vi "StressDist_equivalent.vi"(7 "Corrigido":bool, 8 "Error In":errorcluster, 11 "main_FGV_data":T1={"pipe_properties"={"out_radius"=0.0, "in_radius"=0.0, "out_diameter"=0.0, "in_diameter"=0.0, "thickness"=0.0, "inertia"=0.0, "area"=0.0}, "DirPath"=path "L:/Documentos/00 SERVIÇOS/Tensão residual/Olapa 10-2017/Dados/Primeira Seção/Furos", "DirReport"=path "L:/Documentos/00 SERVIÇOS/Tensão residual/Olapa 10-2017/RelatóriosOlapa/Teste", "Points"=[], "ovalization_data"={"AngOval"=[0.0, 60.0, 120.0, 22.5, 45.0, 67.5, 90.0, 112.5, 135.0, 157.5, 180.0], "OvalDiam"=[324.25, 324.6, 324.55, 324.25, 324.55, 324.65, 324.6, 324.65, 324.55, 324.5, 324.4], "Plots"={"Ref"={"X"=[], "Y"=[]}, "Elipse"={"X"=[], "Y"=[]}, "Points"={"X"=[], "Y"=[]}}, "Ampliation"=100.0, "Results"={"MD"=0.0, "mD"=0.0, "Dmed"=0.0, "Oval"=0.0, "ang"=0.0, "X0"=0.0, "Y0"=0.0}}, "StressDist_data"={"Long"={"Plot"=[], "Fit"=[], "ColorMap"=[], "Data"=[], "peirce_data"={"Plot"=[], "Index removidos"=[]}}, "Circ"={"Plot"=[], "Fit"=[], "ColorMap"=[], "Data"=[], "peirce_data"={"Plot"=[], "Index removidos"=[]}}, "Shear"={"Plot"=[], "Fit"=[], "ColorMap"=[], "Data"=[], "peirce_data"={"Plot"=[], "Index removidos"=[]}}, "Equivalent"={"Plot"=[], "Fit"=[], "ColorMap"=[], "Data"=[], "peirce_data"={"Plot"=[], "Index removidos"=[]}}}, "pressure_data"={"Pressure"=[], "StressCircOval"=[], "StressCirc"=[], "StressLong"=[], "Plot"=[], "Angle"=[]}}) -> (0 "Error Out":errorcluster, 3 "main_FGV_data-out":T1={"pipe_properties"={"out_radius"=0.0, "in_radius"=0.0, "out_diameter"=0.0, "in_diameter"=0.0, "thickness"=0.0, "inertia"=0.0, "area"=0.0}, "DirPath"=path "L:/Documentos/00 SERVIÇOS/Tensão residual/Olapa 10-2017/Dados/Primeira Seção/Furos", "DirReport"=path "L:/Documentos/00 SERVIÇOS/Tensão residual/Olapa 10-2017/RelatóriosOlapa/Teste", "Points"=[], "ovalization_data"={"AngOval"=[0.0, 60.0, 120.0, 22.5, 45.0, 67.5, 90.0, 112.5, 135.0, 157.5, 180.0], "OvalDiam"=[324.25, 324.6, 324.55, 324.25, 324.55, 324.65, 324.6, 324.65, 324.55, 324.5, 324.4], "Plots"={"Ref"={"X"=[], "Y"=[]}, "Elipse"={"X"=[], "Y"=[]}, "Points"={"X"=[], "Y"=[]}}, "Ampliation"=100.0, "Results"={"MD"=0.0, "mD"=0.0, "Dmed"=0.0, "Oval"=0.0, "ang"=0.0, "X0"=0.0, "Y0"=0.0}}, "StressDist_data"={"Long"={"Plot"=[], "Fit"=[], "ColorMap"=[], "Data"=[], "peirce_data"={"Plot"=[], "Index removidos"=[]}}, "Circ"={"Plot"=[], "Fit"=[], "ColorMap"=[], "Data"=[], "peirce_data"={"Plot"=[], "Index removidos"=[]}}, "Shear"={"Plot"=[], "Fit"=[], "ColorMap"=[], "Data"=[], "peirce_data"={"Plot"=[], "Index removidos"=[]}}, "Equivalent"={"Plot"=[], "Fit"=[], "ColorMap"=[], "Data"=[], "peirce_data"={"Plot"=[], "Index removidos"=[]}}}, "pressure_data"={"Pressure"=[], "StressCircOval"=[], "StressCirc"=[], "StressLong"=[], "Plot"=[], "Angle"=[]}})   [LabVIEW 2016]
uses:
  MainFGV/main_FGV_data.ctl
  MainFGV/pipe_properties.ctl
  StressCalculations/point_data.ctl
  Ovalization/ovalization_data.ctl
  StressDist_data.ctl
  StressDist_single_data.ctl
  Peirce/peirce_data.ctl
  Pressure/pressure_data.ctl
  StressDist_types.ctl
  Report/report_mods.ctl
panel:
  out "EquiStressCM":dbl[][](graph)
  out "EquiStress":cluster{"X":dbl[], "Y":dbl[]}[](graph) caption="Ovalização"
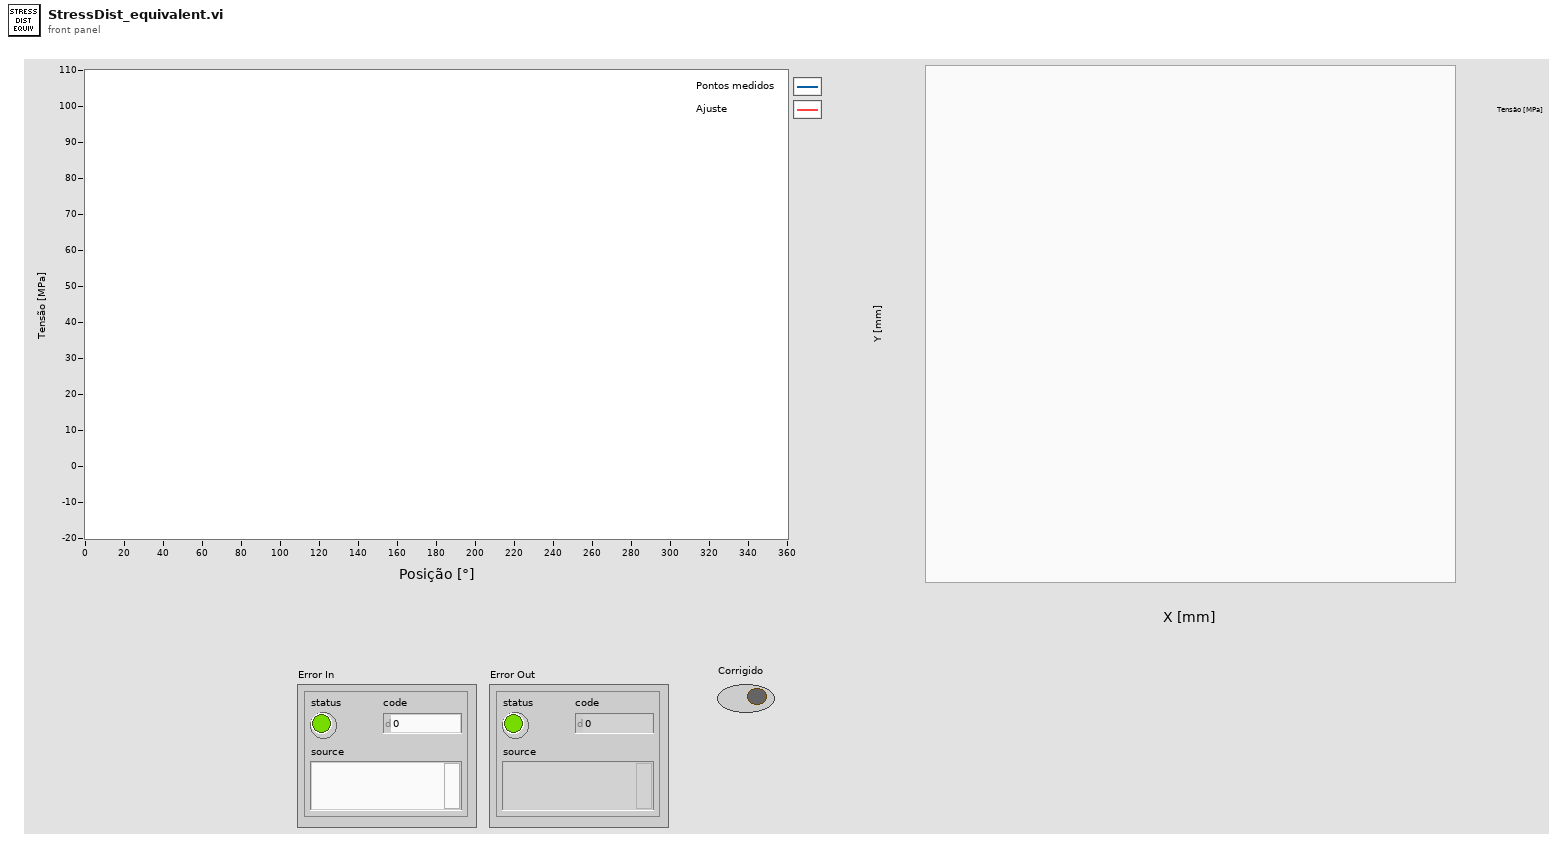
[diagram p1: front panel]
types:
  T1 = typedef "main_FGV_data.ctl" = cluster{"pipe_properties":T2, "DirPath":path, "DirReport":path, "Points":T3[], "ovalization_data":T4, "StressDist_data":T5, "pressure_data":T8}
  T2 = typedef "pipe_properties.ctl" = cluster{"out_radius":dbl, "in_radius":dbl, "out_diameter":dbl, "in_diameter":dbl, "thickness":dbl, "inertia":dbl, "area":dbl}
  T3 = typedef "point_data.ctl" = cluster{"LongStress":dbl, "CircStress":dbl, "ShearStress":dbl, "Pressure":dbl, "Angle":dbl, "Thickness":dbl, "HoleDiam":dbl, "EquiStress":dbl, "S1":dbl, "S2":dbl, "Beta":dbl}
  T4 = typedef "ovalization_data.ctl" = cluster{"AngOval":dbl[], "OvalDiam":dbl[], "Plots":cluster{"Ref":cluster{"X":dbl[], "Y":dbl[]}, "Elipse":cluster{"X":dbl[], "Y":dbl[]}, "Points":cluster{"X":dbl[], "Y":dbl[]}}, "Ampliation":dbl, "Results":cluster{"MD":dbl, "mD":dbl, "Dmed":dbl, "Oval":dbl, "ang":dbl, "X0":dbl, "Y0":dbl}}
  T5 = typedef "StressDist_data.ctl" = cluster{"Long":T6, "Circ":T6, "Shear":T6, "Equivalent":T6}
  T6 = typedef "StressDist_single_data.ctl" = cluster{"Plot":cluster{"Angle":dbl[], "Stress":dbl[]}[], "Fit":dbl[], "ColorMap":dbl[][], "Data":string[][], "peirce_data":T7}
  T7 = typedef "peirce_data.ctl" = cluster{"Plot":cluster{"Array":dbl[], "Array":dbl[]}[], "Index removidos":i32[]}
  T8 = typedef "pressure_data.ctl" = cluster{"Pressure":dbl[], "StressCircOval":dbl[], "StressCirc":dbl[], "StressLong":dbl[], "Plot":cluster{"Angle":dbl[], "Stress":dbl[]}[], "Angle":dbl[]}
  T9 = typedef "report_mods.ctl" = enum16{"Init", "Table", "Graph", "TablefromGraph", "End"}
  T10 = typedef "StressDist_types.ctl" = enum16{"Long", "Circ", "Shear", "Equivalent"}
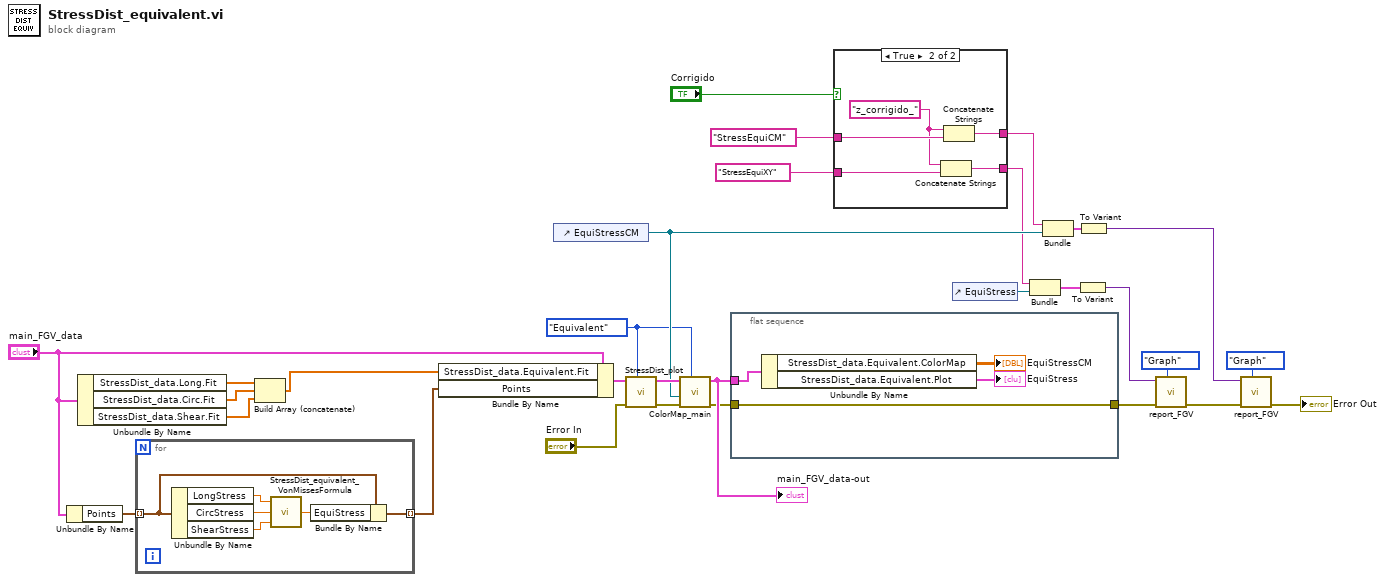
[diagram p0: block diagram]
diagram:
  w10 = StressDist_types."Equivalent" ("StressDist_types")
  n1 = Unbundle By Name("main_FGV_data") -> ("Points"=w4:T3[])
  n2 = Unbundle By Name("main_FGV_data") -> ("StressDist_data.Long.Fit"=w9:dbl[], "StressDist_data.Circ.Fit"=w8:dbl[], "StressDist_data.Shear.Fit"=w7:dbl[])
  n3 = for {
    tunnel: w4 -> [w32] mode=indexing
    tunnel: [w31] -> w3 mode=indexing
    n4 = Unbundle By Name(w32) -> ("LongStress"=w36:dbl, "CircStress"=w35:dbl, "ShearStress"=w34:dbl)
    n5 = call "StressDist_equivalent_VonMissesFormula.vi"("Sshear"=w34, "Scirc"=w35, "Slong"=w36) -> ("Sequi"=w33:dbl)
    n6 = Bundle By Name(cluster=w32, "EquiStress"=w33) -> (w31:T3)
  }
  n7 = Build Array (concatenate)(w9, w8, w7) -> (w6:dbl[])
  n8 = Bundle By Name(cluster="main_FGV_data", "StressDist_data.Equivalent.Fit"=w6, "Points"=w3) -> (w25:T1)
  n9 = control-ref of="EquiStressCM"() -> (w17:refnum<vi>)
  n10 = call "StressDist_plot.vi"("StressDist_types"=w10, "Error In"="Error In", "main_FGV_data"=w25) -> ("Error Out"=w24:errorcluster, "main_FGV_data-out"=w23:T1)  [unwired: 7 in]
  n11 = call "ColorMap_main.vi"("StressDist_types"=w10, "Error In"=w24, "RefCM"=w17, "main_FGV_data"=w23) -> ("Error Out"=w11:errorcluster, "main_FGV_data-out"=w12:T1)  [unwired: 6 in]
  "main_FGV_data-out" <- w12
  n12 = flat-sequence {
    tunnel: w12 -> [w40]
    tunnel: w11 -> [w38]
    tunnel: [w38] -> w29
    frame #0 {
      n13 = Unbundle By Name(w40) -> ("StressDist_data.Equivalent.ColorMap"=→"EquiStressCM":dbl[][], "StressDist_data.Equivalent.Plot"=→"EquiStress":cluster{"Angle":dbl[], "Stress":dbl[]}[])
    }
  }
  n14 = case shown="True" "Corrigido" {
    tunnel: "StressEquiCM" -> [w42 w47]
    tunnel: "StressEquiXY" -> [w41 w45]
    tunnel: [w42 w46] -> w14
    tunnel: [w41 w44] -> w13
    frame False {
    }
    frame True {
      w43 = "z_corrigido_" ("string")
      n15 = Concatenate Strings(w43, w45) -> (w44:string)
      n16 = Concatenate Strings(w43, w47) -> (w46:string)
    }
  }
  n17 = control-ref of="EquiStress"() -> (w26:refnum<vi>)
  n18 = Bundle(w13, "EquiStress"=w26) -> (w28:cluster{string, "EquiStress":refnum<vi>})  [unwired: 1 in]
  n19 = Bundle(w14, "EquiStressCM"=w17) -> (w19:cluster{string, "EquiStressCM":refnum<vi>})  [unwired: 1 in]
  n20 = To Variant(anything=w28) -> (Variant=w27:variant)
  n21 = To Variant(anything=w19) -> (Variant=w18:variant)
  n22 = call "report_FGV.vi"("report_mods"=report_mods."Graph", "Error In"=w29, "Data in"=w27) -> ("Error Out"=w21:errorcluster)  [unwired: 8 in]
  n23 = call "report_FGV.vi"("report_mods"=report_mods."Graph", "Error In"=w21, "Data in"=w18) -> ("Error Out"=→"Error Out":errorcluster)  [unwired: 8 in]
